vi "Builds Updated Callback VI Type.vi"(7 "Owner":refnum<class>, 11 "Builds":T1[](array[typedef])) -> ()   [LabVIEW 2020, in "PicoG-Processor.lvlib"]
uses:
  PicoG-Processor.lvlib
  WebProjectWatcher/Web Build.ctl
  WebProjectWatcher/WebProjectWatcher.lvclass
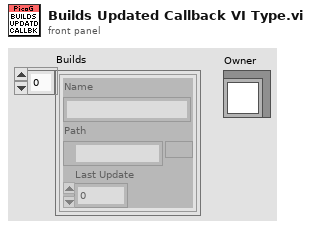
[diagram p1: front panel]
types:
  T1 = typedef "PicoG-Processor.lvlib/WebProjectWatcher.lvclass/Web Build.ctl" = cluster{"Name":string, "Path":path, "Last Update":dbl}
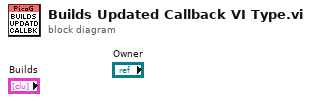
[diagram p0: block diagram]
diagram:
